vi "CreateLogfile.vi"(8 "error in (no error)":errorcluster, 11 "Log File Path":path) -> (0 "error out":errorcluster)   [LabVIEW 2013]
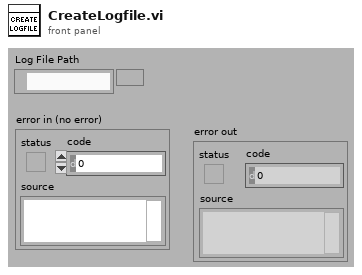
[diagram p1: front panel]
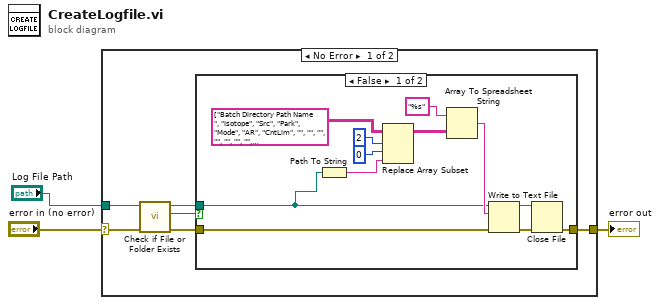
[diagram p0: block diagram]
diagram:
  n1 = case shown="No Error" "error in (no error)" {
    selector: "error in (no error)" -> [w6 w23]
    tunnel: [w4 w23] -> w2
    tunnel: "Log File Path" -> [w5 _]
    frame No Error {
      n2 = call <vilib>:"Check if File or Folder Exists.vi"("error in (no error)"=w6, "path"=w5) -> ("error out"=w8:errorcluster, "file or folder exists?"=w7:bool, "dup path"=w9:path)  [unwired: 7 out]
      n3 = case shown="False" w7 {
        tunnel: w9 -> [w11 _]
        tunnel: w8 -> [w18 w22]
        tunnel: [w19 w22] -> w4
        frame False {
          n4 = Path To String(path=w11) -> (string=w10:string)
          n5 = Replace Array Subset(array=string[][] [["Batch Directory Path Name                                     ", "Isotope", "Src", "Park", "Mode", "AR", "CntLim", "", "", "", "", "", "", "", ""], ["========================================================", "=======", "===", "====", "====", "==", "======", "", "", "", "", "", "", "", ""], ["File Name", "14C", "SNICS", "0", "nrm", "no", "100", "", "", "", "", "", "", "", ""], ["", "", "", "", "", "", "", "", "", "", "", "", "", "", ""], ["Run Completion Time       ", "Pos", "Meas", "Sample Name", "Num", "Cycles", "le12C      ", "le13C      ", "he12C      ", "he13C      ", "CntTotH", "CntTotS", "CntTotGT", "13/12he    ", "14/12he    "], ["========================", "===", "====", "===========", "===", "======", "===========", "===========", "===========", "===========", "=======", "=======", "========", "===========", "==========="]] ("Header1"), new element=w10, index (row)=2, index (col)=0 ("disabled index (col)")) -> (w15:string[][])
          n6 = Array To Spreadsheet String(array=w15, 3:"%s" ("format string")) -> (spreadsheet string=w12:string)  [unwired: 1 out]
          n7 = Write to Text File(file (use dialog)=w11, text=w12, error in=w18) -> (refnum out=w21:refnum<file>, error out=w20:errorcluster)  [unwired: 2 out]
          n8 = Close File(refnum=w21, error in=w20) -> (error out=w19:errorcluster)  [unwired: 1 out]
        }
        frame True {
        }
      }
    }
    frame Error {
    }
  }
  "error out" <- w2
